vi "IRH3T Stand Alone Tester.vi"() -> ()   [LabVIEW 2013]
uses:
  Classes/OSSP_Problem.lvclass
  GA/Controls/Scheduler Type.ctl
  Initial Construction Heuristic.ctl
  Classes/OSSP_Problem.lvclass/OSSP_Problem.ctl
  Classes/Scheduler_Class/Operation to Machine Job Tuple.vi
  <vilib>/dlg_ctls.llb/Space Constant.vi
  Classes/Scheduler_Class/NonDelay Scheduler/Non Delay Scheduler Engine.vi
  Classes/Scheduler_Class/Prins FIFO Scheduler Methods and Controls/Prins FIFO Scheduler.vi
  Classes/Scheduler_Class/Prins FIFO Scheduler Methods and Controls/Methods/Calculate Final Completion Times of Jobs.vi
  GA/SubVIS/Calcualte General Tardiness.vi
  LPTSequenceBulilder.vi
  SPTSequenceBulilder.vi
  EDDSequenceBulilder.vi
  Classes/Scheduler_Class/Prins FIFO Scheduler Methods and Controls/Methods/UpdateMachineGaps.vi
  Classes/Scheduler_Class/Prins FIFO Scheduler Methods and Controls/Methods/UpdateJobGaps.vi
  Classes/Scheduler_Class/Prins FIFO Scheduler Methods and Controls/Methods/Find Intersecting Gaps.vi
panel:
  out "Due Dates":bool[](array[boolean])
  out "IRH3T Schedule Out":u16[](array[numeric])
  out "IRH3T (Reordered) Schedule Out":u16[](array[numeric])
  out "Total Tardiness":u16
  in  "Problem Type":enum16{"Taillard", "Brucker", "Gueret Prins"}(ring)=enum."Brucker"
  in  "Instance Number for Taillard":dbl
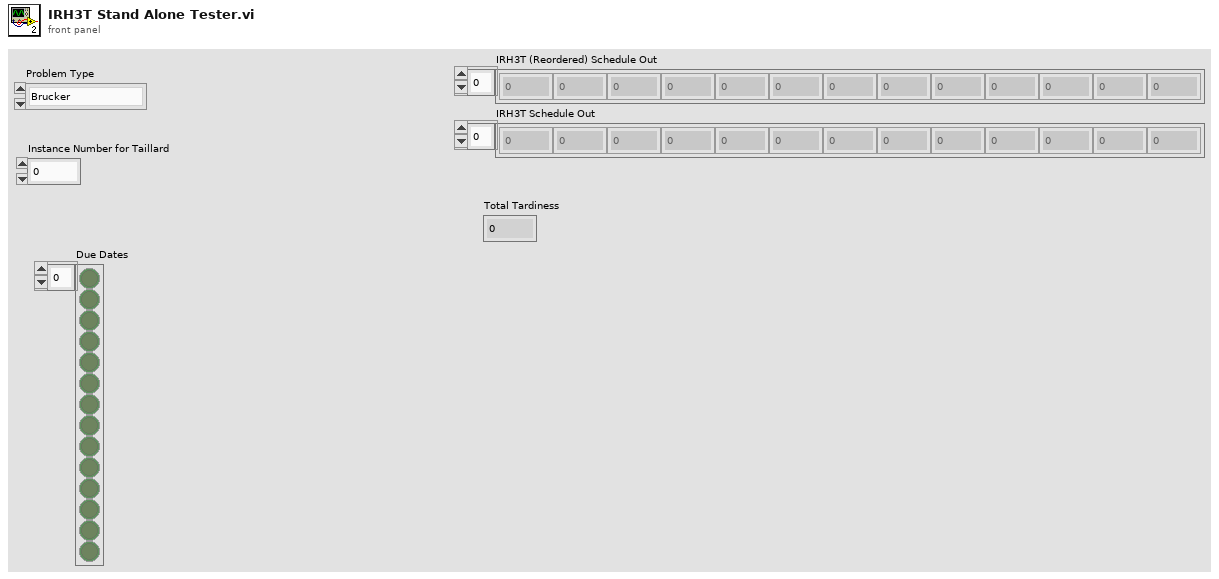
[diagram p1: front panel]
types:
  T1 = typedef "Initial Construction Heuristic.ctl" = enum16{"LPT", "SPT", "EDD"}
  T2 = typedef "Scheduler Type.ctl" = enum16{"Non Delay Scheduler", "GT Active Scheduler", "My Faulty Scheduler", "Prins FIFO Scheduler", "SemiActive Scheduler"}
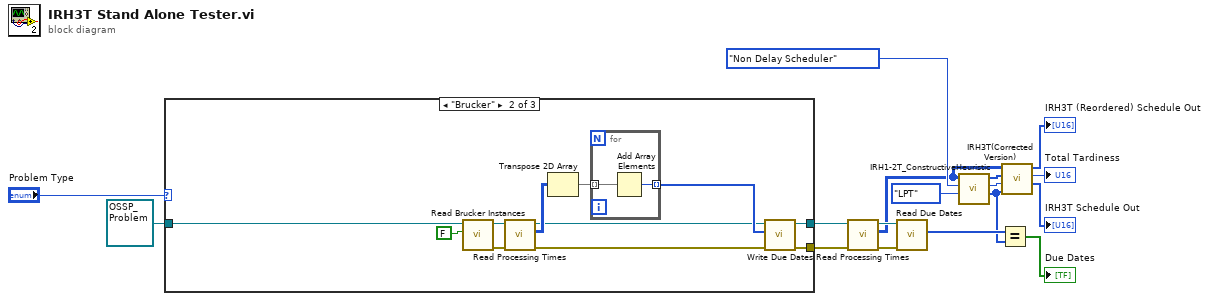
[diagram p0: block diagram]
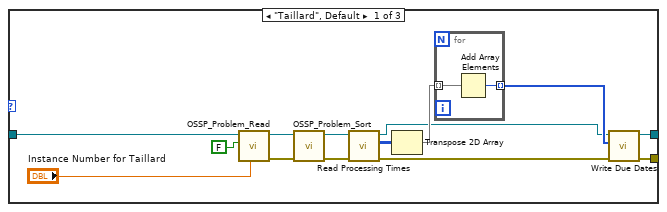
[diagram p2: hidden frame]
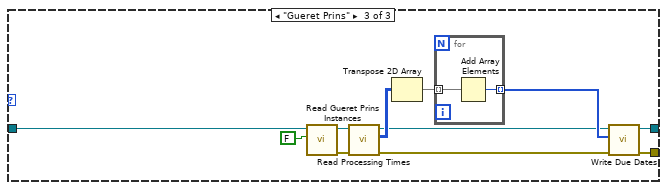
[diagram p3: hidden frame]
diagram:
  n1 = case shown="\"Brucker\"" "Problem Type" {
    tunnel: refnum<class "OSSP_Problem.lvclass"> refnum ("OSSP_Problem.lvclass") -> [w31 w44 w57]
    tunnel: [w24 w39 w52] -> w5
    tunnel: [w23 w40 w53] -> w4
    frame "Taillard", Default {
      n2 = call "OSSP_Problem_Read.vi"("Instance Number"="Instance Number for Taillard", "Auto Mode"=FALSE, "OSSP_Problem.lvclass In"=w31) -> ("error out"=w28:errorcluster, "OSSP_Problem.lvclass Out"=w29:refnum<class "OSSP_Problem.lvclass">)  [unwired: 7 in]
      n3 = call "OSSP_Problem_Sort.vi"("error in (no error)"=w28, "OSSP_Problem.lvclass In"=w29) -> ("error out"=w26:errorcluster, "OSSP_Problem.lvclass Out"=w25:refnum<class "OSSP_Problem.lvclass">)  [unwired: 8 in]
      n4 = call "Read Processing Times.vi"("error in (no error)"=w26, "OSSP_Problem in"=w25) -> ("error out"=w18:errorcluster, "Processing Times"=w21:u16[][], "OSSP_Problem out"=w19:refnum<class "OSSP_Problem.lvclass">)  [unwired: 7 in]
      n5 = Transpose 2D Array(2D array=w21) -> (transposed array=w22:u16[][])
      n6 = for {
        tunnel: w22 -> [w33] mode=indexing
        tunnel: [w32] -> w20 mode=indexing
        n7 = Add Array Elements(numeric array=w33) -> (sum=w32:u16)
      }
      n8 = call "Write Due Dates.vi"("error in (no error)"=w18, "Due Dates"=w20, "OSSP_Problem in"=w19) -> ("error out"=w23:errorcluster, "OSSP_Problem out"=w24:refnum<class "OSSP_Problem.lvclass">)  [unwired: 7 in]
    }
    frame "Brucker" {
      n9 = call "Read Brucker Instances.vi"("Auto Mode"=FALSE, "OSSP_Problem in"=w44) -> ("error out"=w41:errorcluster, "OSSP_Problem out"=w42:refnum<class "OSSP_Problem.lvclass">)  [unwired: 8 in]
      n10 = call "Read Processing Times.vi"("error in (no error)"=w41, "OSSP_Problem in"=w42) -> ("error out"=w34:errorcluster, "Processing Times"=w37:u16[][], "OSSP_Problem out"=w35:refnum<class "OSSP_Problem.lvclass">)  [unwired: 7 in]
      n11 = Transpose 2D Array(2D array=w37) -> (transposed array=w38:u16[][])
      n12 = for {
        tunnel: w38 -> [w46] mode=indexing
        tunnel: [w45] -> w36 mode=indexing
        n13 = Add Array Elements(numeric array=w46) -> (sum=w45:u16)
      }
      n14 = call "Write Due Dates.vi"("error in (no error)"=w34, "Due Dates"=w36, "OSSP_Problem in"=w35) -> ("error out"=w40:errorcluster, "OSSP_Problem out"=w39:refnum<class "OSSP_Problem.lvclass">)  [unwired: 7 in]
    }
    frame "Gueret Prins" {
      n15 = call "Read Gueret Prins Instances.vi"("Auto Mode"=FALSE, "OSSP_Problem in"=w57) -> ("error out"=w54:errorcluster, "OSSP_Problem out"=w55:refnum<class "OSSP_Problem.lvclass">)  [unwired: 8 in]
      n16 = call "Read Processing Times.vi"("error in (no error)"=w54, "OSSP_Problem in"=w55) -> ("error out"=w47:errorcluster, "Processing Times"=w50:u16[][], "OSSP_Problem out"=w48:refnum<class "OSSP_Problem.lvclass">)  [unwired: 7 in]
      n17 = Transpose 2D Array(2D array=w50) -> (transposed array=w51:u16[][])
      n18 = for {
        tunnel: w51 -> [w59] mode=indexing
        tunnel: [w58] -> w49 mode=indexing
        n19 = Add Array Elements(numeric array=w59) -> (sum=w58:u16)
      }
      n20 = call "Write Due Dates.vi"("error in (no error)"=w47, "Due Dates"=w49, "OSSP_Problem in"=w48) -> ("error out"=w53:errorcluster, "OSSP_Problem out"=w52:refnum<class "OSSP_Problem.lvclass">)  [unwired: 7 in]
    }
  }
  n21 = call "Read Processing Times.vi"("error in (no error)"=w4, "OSSP_Problem in"=w5) -> ("error out"=w15:errorcluster, "Processing Times"=w10:u16[][], "OSSP_Problem out"=w16:refnum<class "OSSP_Problem.lvclass">)  [unwired: 7 in]
  n22 = call "Read Due Dates.vi"("error in (no error)"=w15, "OSSP_Problem in"=w16) -> ("Due Dates"=w3:u16[])  [unwired: 7 in, 2 out]
  n23 = call "IRH1-2T_ConstructiveHeuristic.vi"("Initial Construction Heursitic"=Initial_Construction_Heuristic."LPT", "Scheduler"=Scheduler_Type."Non Delay Scheduler", "Proocessing Times MxJ"=w10) -> ("Due Dates"=w2:u16[], "Total Tardiness"=w9:u16, "IRH2T Schedule Out"=w11:u16[])  [unwired: 6 in]
  n24 = Equal?(x=w3, y=w2) -> (x = y?=→"Due Dates":bool[])
  n25 = call "IRH3T(Corrected Version).vi"("Due Dates"=w2, "Initial Tardiness"=w9, "Schedule 2B Improved"=w11, "Proocessing Times  (Machines x Jobs)"=w10) -> ("IRH3T Schedule Out"=→"IRH3T Schedule Out":u16[], "Total Tardiness"=→"Total Tardiness":u16, "IRH3T (Reordered) Schedule Out"=→"IRH3T (Reordered) Schedule Out":u16[])  [unwired: 5 in]
